vi "Delete QPD outside region(SubVI).vi"(9 "Position Array In":dbl[](array[numeric]), 11 "QPD signal In":dbl[](array[numeric])) -> (1 "Position Array Out":dbl[](array[numeric]), 3 "QPD signal Out":dbl[](array[numeric]))   [LabVIEW 2014]
doc: "This VI deletes the region outside of the QPD max value and min value.\nClean up the signal for fitting."
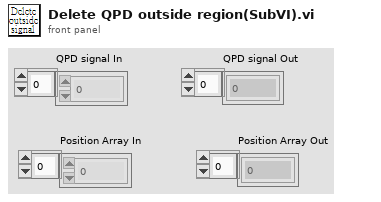
[diagram p1: front panel]
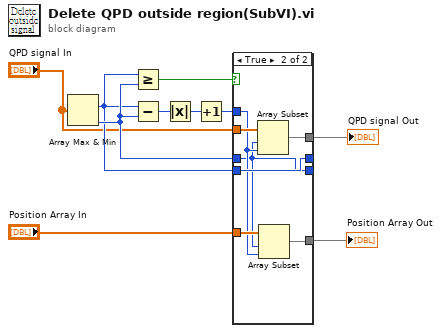
[diagram p0: block diagram]
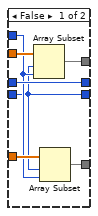
[diagram p2: hidden frame]
diagram:
  n1 = Array Max & Min(array="QPD signal In") -> (max index (indices)=w6:i32, min index (indices)=w7:i32)  [unwired: 2 out]
  n2 = Greater Or Equal?(x=w6, y=w7) -> (x >= y?=w4:bool)
  n3 = Subtract(x=w6, y=w7) -> (x-y=w1:i32)
  n4 = Absolute Value(x=w1) -> (abs(x)=w8:i32)
  n5 = Increment(x=w8) -> (x+1=w9:i32)
  n6 = case shown="True" w4 {
    tunnel: w6 -> [w12 w22]
    tunnel: w7 -> [w15 w18]
    tunnel: "QPD signal In" -> [w17 w24]
    tunnel: w9 -> [w13 w19]
    tunnel: [w16 w23] -> w10
    tunnel: [w15 w22] -> _
    tunnel: [w12 w18] -> _
    tunnel: "Position Array In" -> [w14 w21]
    tunnel: [w11 w20] -> w2
    frame False {
      n7 = Array Subset(array=w17, index=w12, length=w13) -> (w16:dbl[])
      n8 = Array Subset(array=w14, index=w12, length=w13) -> (w11:dbl[])
    }
    frame True {
      n9 = Array Subset(array=w24, index=w18, length=w19) -> (w23:dbl[])
      n10 = Array Subset(array=w21, index=w18, length=w19) -> (w20:dbl[])
    }
  }
  "QPD signal Out" <- w10
  "Position Array Out" <- w2
